vi "4_Tx_DSB_AM.vi"() -> ()   [LabVIEW 2022 SP3]
uses:
  <instrlib>/niUSRP/niUSRP Write Tx Data (CDB WDT).vi
panel:
  out "Modulated wave":waveform(dbl)(graph)
  out "Carrier":dynamicdata(graph)
  out "Message":dynamicdata(graph)
  in  "Am":dbl=1.0 caption="Amplitude"
  in  "Ac":dbl=1.0 caption="Amplitude"
  in  "stop":bool
  in  "active antenna":string
  in  "gain":dbl format="%#_6f"
  in  "carrier frequency":dbl=100000.0 format="%#_6p"
  in  "IQ rate":dbl=100000.0 format="%#_6p"
  in  "device names":refnum<k15>
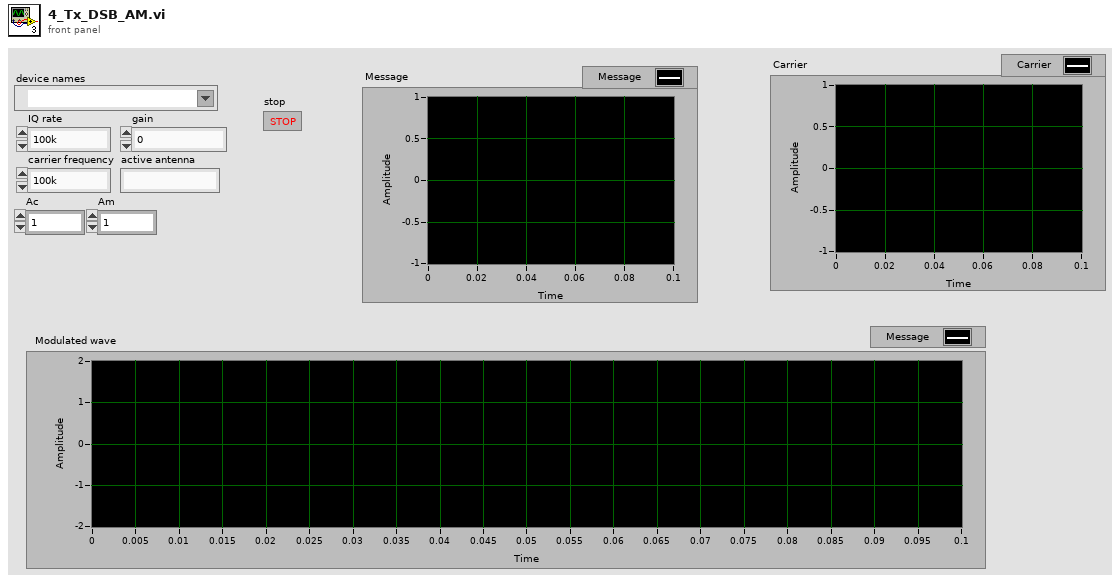
[diagram p1: front panel]
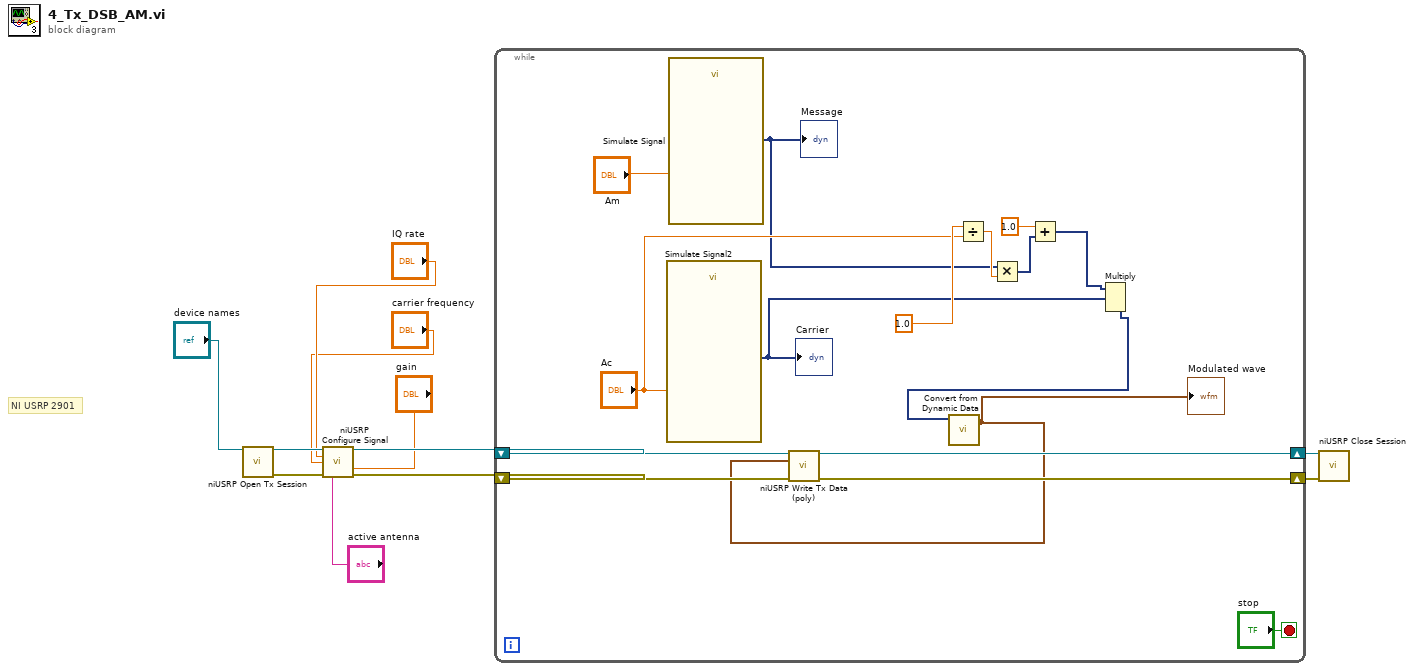
[diagram p0: block diagram]
diagram:
  # "NI USRP 2901"
  n1 = call <instrlib>:"niUSRP Open Tx Session.vi"("device names"="device names") -> ("session handle out"=w10:refnum<k15>, "error out"=w9:errorcluster)  [unwired: 13 in]
  n2 = call <instrlib>:"niUSRP Configure Signal.vi"("session handle"=w10, "IQ rate"="IQ rate", "carrier frequency"="carrier frequency", "gain"="gain", "error in (no error)"=w9, "active antenna"="active antenna") -> ("session handle out"=w8:refnum<k15>, "error out"=w7:errorcluster)  [unwired: 5 in, 3 out]
  n3 = while {
    shift-right: [w25] -> w6
    shift-left: w8 -> [w27]
    shift-right: [w24] -> w5
    shift-left: w7 -> [w26]
    stop <- "stop" stop-if-true
    n4 = call "Simulate Signal2"("Amplitude"="Ac") -> ("Carrier"=w14:dynamicdata)  [unwired: 13 in, 1 out]
    "Carrier" <- w14
    n5 = call "Simulate Signal"("Amplitude"="Am") -> ("Message"=w18:dynamicdata)  [unwired: 13 in, 1 out]
    "Message" <- w18
    n6 = Divide(x=1.0, y="Ac") -> (x/y=w19:dbl)
    n7 = Multiply(x=w18, y=w19) -> (x*y=w16:dynamicdata)
    n8 = Add(x=1.0, y=w16) -> (x+y=w15:dynamicdata)
    n9 = Multiply(1:w14, 2:w15) -> (0:w13:dynamicdata)  [unwired: 1 in, 1 out]
    n10 = call "Convert from Dynamic Data"("Dynamic Data Type"=w13) -> ("Waveform"=w12:waveform(dbl))  [unwired: 3 in]
    "Modulated wave" <- w12
    n11 = call-poly <instrlib>:"niUSRP Write Tx Data (poly).vi"("session handle"=w27, "data"=w12, "error in (no error)"=w26) -> ("session handle out"=w25:refnum<k15>, "error out"=w24:errorcluster)  [unwired: 11 in]
  }
  n12 = call <instrlib>:"niUSRP Close Session.vi"("session handle"=w6, "error in (no error)"=w5) -> ()  [unwired: 13 in, 1 out]
